vi "Spectrograph_acceptCommand_setupSpectrograph.vi"(8 "error in (no error)":errorcluster, 11 "command_setupSpectrograph_Ctl":T1) -> (0 "error out":errorcluster, 2 "function return":i32, 3 "command_setupSpectrograph_Ctl out":T1)   [LabVIEW 2016, in "SALLV_Spectrograph.lvlib"]
doc: "int Spectrograph_shm_acceptCommand_setupSpectrographLV(Spectrograph_command_setupSpectrographLV *command_setupSpectrograph_Ctl );"
uses:
  SALLV_Spectrograph.lvlib
  DataTypes/command_setupSpectrograph.ctl
  SALLV_Spectrograph.so
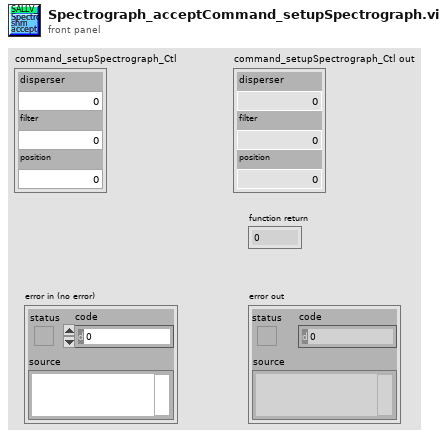
[diagram p1: front panel]
types:
  T1 = typedef "SALLV_Spectrograph.lvlib/command_setupSpectrograph.ctl" = cluster{"disperser":i32, "filter":i32, "position":dbl}
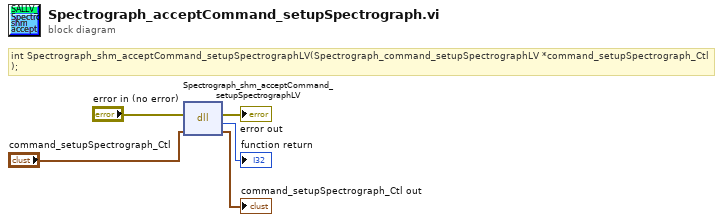
[diagram p0: block diagram]
diagram:
  # "int Spectrograph_shm_acceptCommand_setupSpectrographLV(Spectrograph_command_setupSpectrographLV *command_setupSpectrograph_Ctl );"
  n1 = dll-call lib="home/harini/TCS/SALLV_Spectrograph/SALLV_Spectrograph.*" fn="Spectrograph_shm_acceptCommand_setupSpectrographLV"(error in="error in (no error)", "command_setupSpectrograph_Ctl"="command_setupSpectrograph_Ctl") -> (error out=→"error out":errorcluster, →"function return":i32, "command_setupSpectrograph_Ctl"=→"command_setupSpectrograph_Ctl out":T1)  [unwired: 2 in, 1 out]
